vi "Control.vi"(1 "Page":i8 min=0 max=3 step=1, 2 "Error":bool, 3 "Write":bool, 4 "Addr":i8 min=0 max=15 step=1) -> (0 "Control Byte":u32 format="%x")   [LabVIEW 2012]
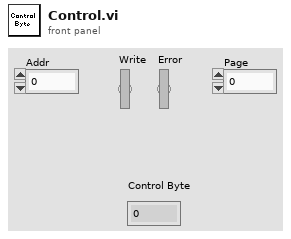
[diagram p1: front panel]
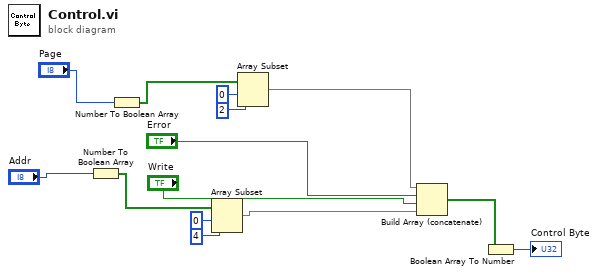
[diagram p0: block diagram]
diagram:
  n1 = Number To Boolean Array(number="Addr") -> (Boolean array=w13:bool[])
  n2 = Number To Boolean Array(number="Page") -> (Boolean array=w7:bool[])
  n3 = Array Subset(array=w13, index=0, length=4) -> (w4:bool[])
  n4 = Array Subset(array=w7, index=0, length=2) -> (w1:bool[])
  n5 = Build Array (concatenate)(w1, "Error", "Write", w4) -> (w6:bool[])
  n6 = Boolean Array To Number(Boolean array=w6) -> (number=→"Control Byte":u32)
